vi "writeonlycommand(sub).vi"(0 "resourcein":refnum<visa-resource-name>, 1 "Command":dbl, 2 "Commandprefix":string="R0003", 3 "errorin":errorcluster) -> (5 "resourceout":refnum<visa-resource-name>, 6 "errorout":errorcluster)   [LabVIEW 2015]
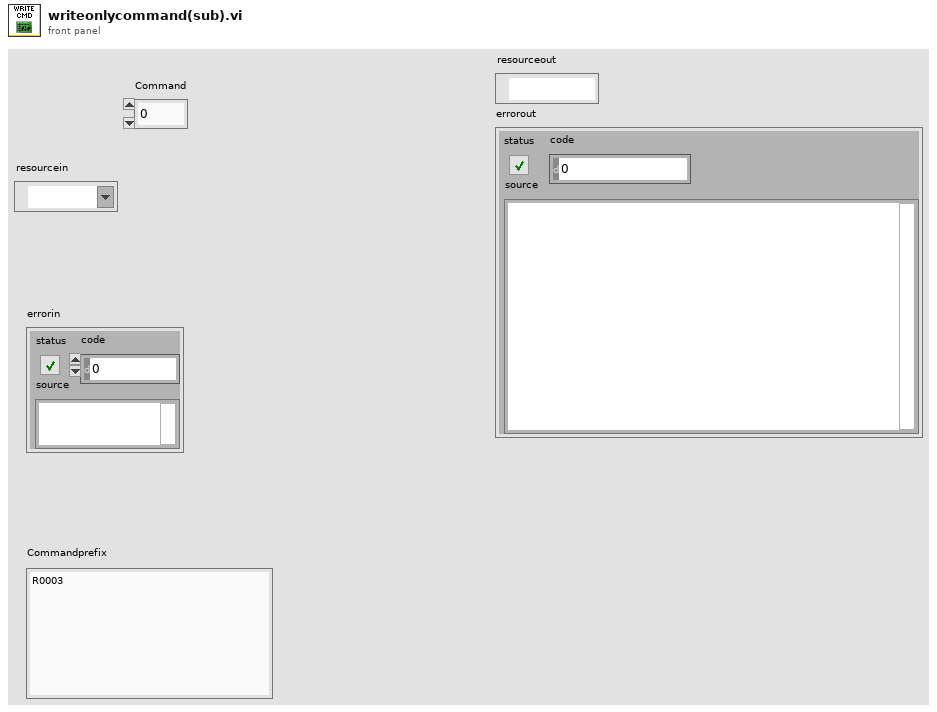
[diagram p1: front panel]
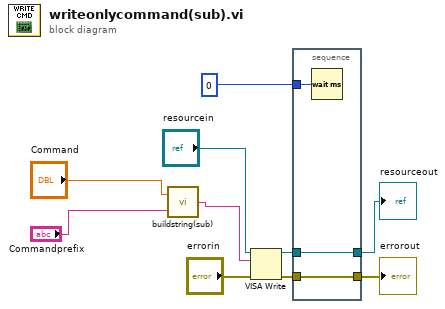
[diagram p0: block diagram]
diagram:
  n1 = call "buildstring(sub).vi"("Prefix"="Commandprefix", "Command"="Command") -> ("Commandstring"=w4:string)
  n2 = VISA Write(VISA resource name="resourcein", write buffer=w4, error in (no error)="errorin") -> (VISA resource name out=w8:refnum<visa-resource-name>, error out=w7:errorcluster)  [unwired: 1 out]
  n3 = stacked-sequence {
    tunnel: w7 -> [w13]
    tunnel: [w13] -> w5
    tunnel: w8 -> [w12]
    tunnel: [w12] -> w6
    tunnel: u32 0 ("readdelay") -> [w11]
    frame #0 {
      n4 = Wait (ms)(milliseconds to wait=w11) -> ()  [unwired: 1 out]
    }
  }
  "resourceout" <- w6
  "errorout" <- w5
